vi "LWXPS_PositionerCorrectorPIDAccelerationFilterGet.vi"(0 "XPS Reference IN":refnum<k24>, 7 "Positioner Name":string, 11 "LabVIEW error IN":errorcluster) -> (3 "XPS Reference OUT":refnum<k24>, 4 "Returned error code":i32, 6 "Filter Control Status":bool, 8 "KD Gain":dbl, 10 "Derivative Filter Cut Off Frequency":dbl, 14 "LabVIEW error OUT":errorcluster, 15 "XPS Error String":string)   [LabVIEW 2014]
uses:
  D:/XPSQ8_LabView_Library/Development/Source/Dll/Newport.XPS.CommandInterface.dll
  Dll/Newport.XPS.CommandInterface.dll
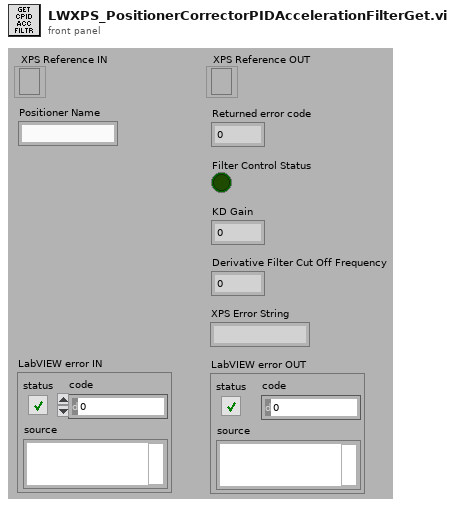
[diagram p1: front panel]
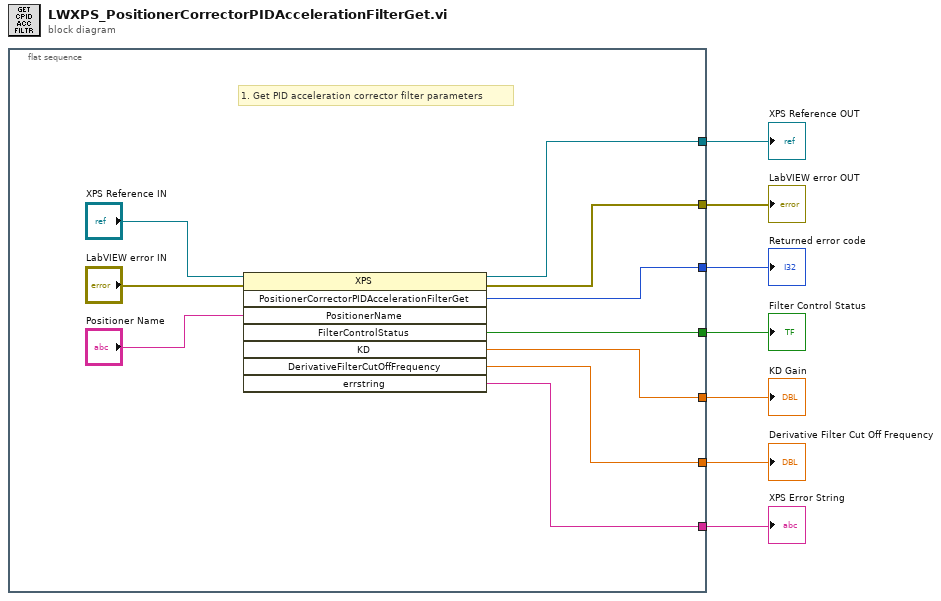
[diagram p0: block diagram]
diagram:
  n1 = flat-sequence {
    tunnel: [w15] -> w7
    tunnel: [w12] -> w6
    tunnel: [w16] -> w5
    tunnel: [w8] -> w2
    tunnel: [w11] -> w4
    tunnel: [w10] -> w3
    tunnel: [w9] -> w1
    frame #0 {
      # "1. Get PID acceleration corrector filter parameters"
      n2 = invoke class="XPS" method="PositionerCorrectorPIDAccelerationFilterGet"(reference="XPS Reference IN", error in="LabVIEW error IN", "PositionerName"="Positioner Name") -> (reference out=w15:refnum<k24>, error out=w12:errorcluster, "PositionerCorrectorPIDAccelerationFilterGet"=w16:i32, "FilterControlStatus"=w8:bool, "KD"=w11:dbl, "DerivativeFilterCutOffFrequency"=w10:dbl, "errstring"=w9:string)  [unwired: 5 in, 1 out]
    }
  }
  "XPS Error String" <- w1
  "XPS Reference OUT" <- w7
  "LabVIEW error OUT" <- w6
  "Returned error code" <- w5
  "KD Gain" <- w4
  "Derivative Filter Cut Off Frequency" <- w3
  "Filter Control Status" <- w2
